vi "FPGA Main Full Compile Test.vi"() -> ()   [LabVIEW 2010]
uses:
  Motor Control/Motor Encoder Global.vi
  Motor Control/Motor Output Global.vi
  Motor Control/Inner Control/Drive Control Global DO NOT MODIFY!.vi
  behaviors/driveable path/drivable paths global.vi
  FPGA Opperation Mode.ctl
panel:
  out "Steering Position":i32
  out "Drive Speed Current":fxp<+/-,18,8> format="%.13g"
  out "Drive Enable":bool
  out "Steering Enable":bool
  out "driveable path lengths":u16[](array[numeric])
  in  "Autonomous Drive Current":fxp<+/-,18,8>
  in  "min obstacle dist":u16
  in  "Enum":T1
  in  "Steering Position Offset":i32
  out "Drive Encoder ft/sec":fxp<+/-,18,8>
  in  "Drive Enable":bool
  in  "Drive Speed Current (1-3.5)":fxp<+/-,18,8>
  in  "Stop":bool
  in  "Steering Proportional Control Feedback Gain":fxp<+/-,20,5>
  in  "Steering Enable":bool
  in  "Steering Position Target":i32
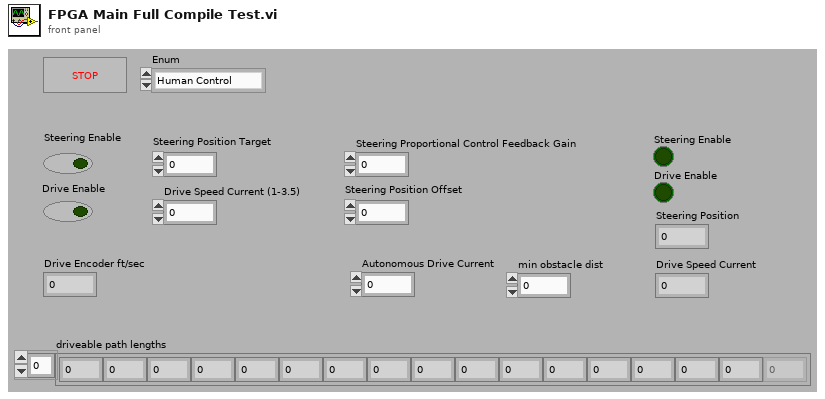
[diagram p1: front panel]
types:
  T1 = typedef "FPGA Opperation Mode.ctl" = enum16{"Human Control", "Autonomous"}
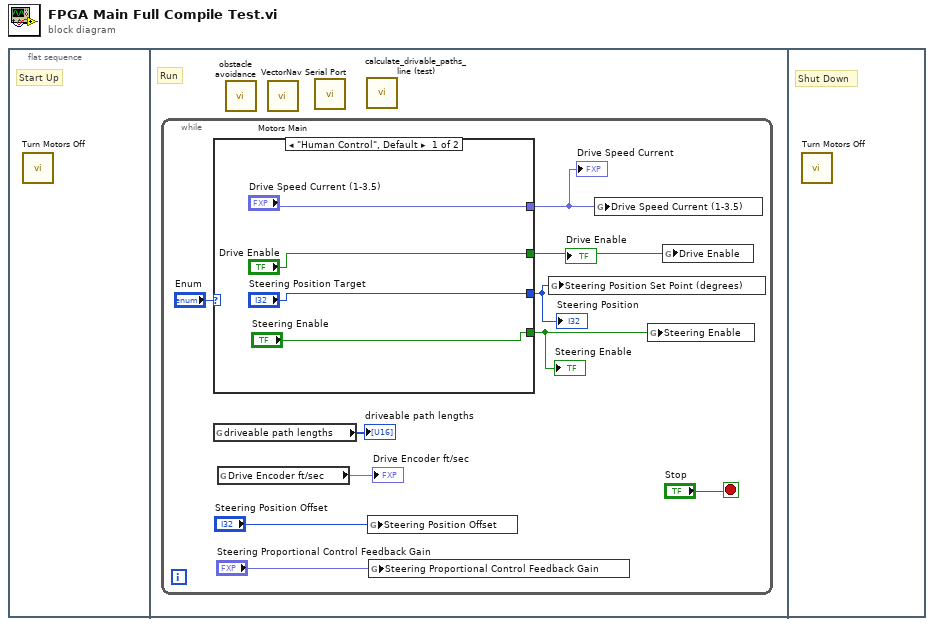
[diagram p0: block diagram]
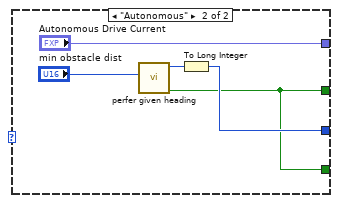
[diagram p2: hidden frame]
diagram:
  n1 = flat-sequence {
    frame #0 {
      # "Start Up"
      n2 = call "Turn Motors Off.vi"() -> ()  [unwired: 1 in]
    }
    frame #1 {
      # "Run"
      n3 = while {
        stop <- "Stop" stop-if-true
        n4 = case shown="\"Human Control\", Default" "Enum" {
          tunnel: ["Steering Position Target" w17] -> w1
          tunnel: ["Drive Enable" w16] -> w6
          tunnel: ["Steering Enable" w16] -> w5
          tunnel: ["Drive Speed Current (1-3.5)" "Autonomous Drive Current"] -> w4
          frame "Human Control", Default {
          }
          frame "Autonomous" {
            n5 = call "perfer given heading.vi"("min obstacle dist"="min obstacle dist") -> ("driveable paths?"=w16:bool, "wheel angle"=w18:i8)  [unwired: 9 in]
            n6 = To Long Integer(number=w18) -> (32bit integer=w17:i32)
          }
        }
        "Steering Enable" <- w5
        "Drive Enable" <- w6
        "Drive Speed Current" <- w4
        "Steering Position" <- w1
        n7 = global read "drivable paths global.vi" "driveable path lengths"() -> (→"driveable path lengths":u16[])
        n8 = global read "Drive Control Global DO NOT MODIFY!.vi" "Drive Encoder ft/sec"() -> (→"Drive Encoder ft/sec":fxp<+/-,18,8>)
        n9 = global write "Motor Encoder Global.vi" "Steering Position Offset"("Steering Position Offset") -> ()
        n10 = global write "Motor Encoder Global.vi" "Steering Proportional Control Feedback Gain"("Steering Proportional Control Feedback Gain") -> ()
        n11 = global write "Motor Encoder Global.vi" "Steering Position Set Point (degrees)"(w1) -> ()
        n12 = global write "Motor Encoder Global.vi" "Drive Speed Current (1-3.5)"(w4) -> ()
        n13 = global write "Motor Output Global.vi" "Steering Enable"(w5) -> ()
        n14 = global write "Motor Output Global.vi" "Drive Enable"(w6) -> ()
      }
      n15 = call "obstacle avoidance.vi"() -> ()  [unwired: 1 in]
      n16 = call "Motors Main.vi"() -> ()  [unwired: 1 in]
      n17 = call "VectorNav Serial Port.vi"() -> ()  [unwired: 12 in]
      n18 = call "calculate_drivable_paths_line (test).vi"() -> ()  [unwired: 1 in]
    }
    frame #2 {
      # "Shut Down"
      n19 = call "Turn Motors Off.vi"() -> ()  [unwired: 1 in]
    }
  }
